vi "datagen 2.vi"() -> ()   [LabVIEW 2020]
uses:
  <vilib>/Graiphic/HAIBAL Deep learning/Source/Layer/Dense/_Controls/dense_param.ctl
  <vilib>/Graiphic/HAIBAL Deep learning/Source/_Controls/activation_enum.ctl
  <vilib>/Graiphic/HAIBAL Deep learning/Source/_Controls/optimizer_param.ctl
  <vilib>/Graiphic/HAIBAL Deep learning/Source/_Controls/optimizer_enum.ctl
  <vilib>/Graiphic/HAIBAL Deep learning/Source/Init/_Controls/Init_Enum.ctl
  <vilib>/Graiphic/HAIBAL Deep learning/Source/Model/Controls/frw_training_mode.ctl
  <vilib>/Graiphic/HAIBAL Deep learning/Source/Layer/Input/_Methods/add_to_graph.vi
  <vilib>/Graiphic/HAIBAL Deep learning/Source/Layer/Dense/_Methods/add_to_graph.vi
  <vilib>/Graiphic/HAIBAL Deep learning/Source/Model/_Methods/summary.vi
  <vilib>/Graiphic/HAIBAL Deep learning/Source/Model/_Methods/mono_input_2d.vi
  <vilib>/Graiphic/HAIBAL Deep learning/Source/Model/_Methods/mono_y_true_2d.vi
  <vilib>/Graiphic/HAIBAL Deep learning/Source/Model/_Methods/backward.vi
  <vilib>/Graiphic/HAIBAL Deep learning/Source/Model/_Methods/get_2d_output_frw.vi
  <vilib>/Graiphic/HAIBAL Deep learning/Source/Layer/Dense/Dense.lvclass
  <vilib>/Graiphic/HAIBAL Deep learning/Source/Model/Model.lvclass
  <vilib>/Graiphic/HAIBAL Deep learning/Source/Layer/Input/Input.lvclass
panel:
  out "Waveform Chart":sgl(graph)
  out "Epoch":i32
  out "Display":cluster{"X":dbl, "Y_True":dbl, "Y_Pred":dbl}[](graph)
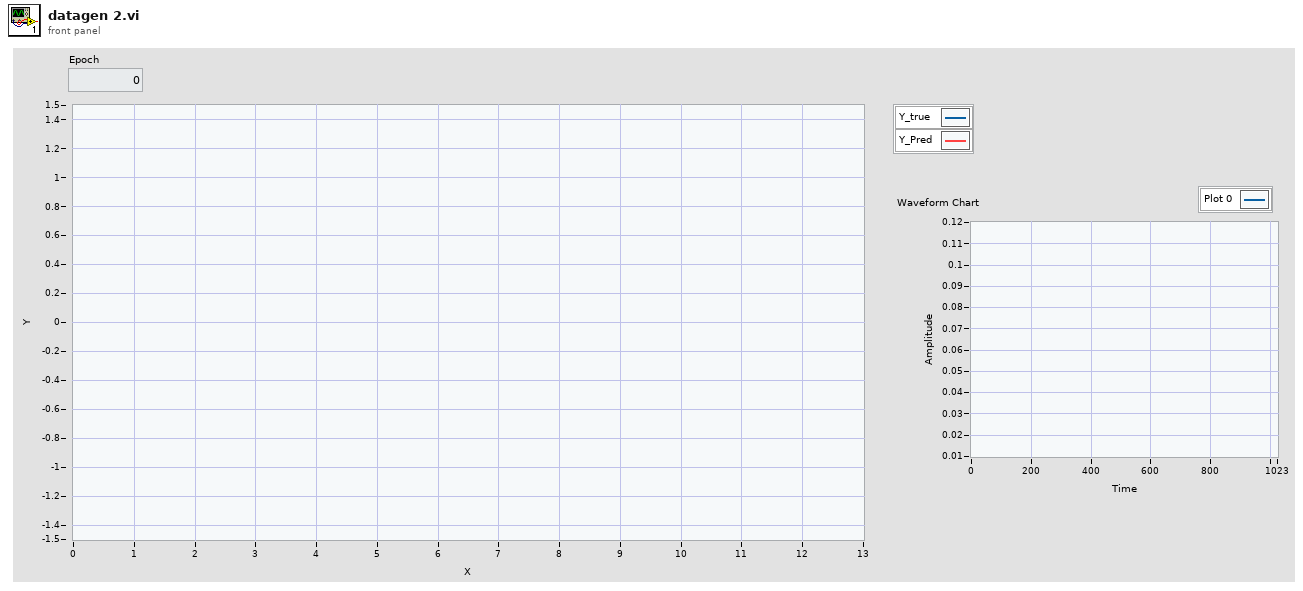
[diagram p1: front panel]
types:
  T1 = typedef "Dense.lvclass/dense_param.ctl" = cluster{"units":i32, "activation":T2, "use_bias?":bool, "optimizer":T3, "weight_initializer":T5, "bias_initializer":T5, "training?":bool, "store?":bool, "update?":bool, "lda_coeff":dbl}
  T2 = typedef "activation_enum.ctl" = enum16{"elu", "exponential", "gelu", "hard_sigmoid", "leaky_relu", "linear", "relu", "selu", "sigmoid", "softmax", "softplus", "softsign", "swish", "tanh", "thresholdedrelu"}
  T3 = typedef "optimizer_param.ctl" = cluster{"algorithm":T4, "learning_rate":sgl, "beta_1":sgl, "beta_2":sgl}
  T4 = typedef "optimizer_enum.ctl" = enum16{"adadelta", "adagrad", "adam", "adamax", "inertia", "nadam", "nesterov", "rmsprop", "sgd"}
  T5 = typedef "Init_Enum.ctl" = enum16{"Constant", "GlorotNormal", "GlorotUniform", "HeNormal", "HeUniform", "Identity", "LeCunNormal", "LeCunUniform", "Ones", "Orthogonal", "RandomNormal", "RandomUniform", "TruncatedNormal", "VarianceScaling", "Zeros"}
  T6 = typedef "frw_training_mode.ctl" = enum16{"Nothing", "Training", "Predict"}
  T7 = typedef "loss_data_cluster.ctl" = cluster{"loss":sgl, "loss_derivate":T8[]}
  T8 = typedef "backward_output_cluster.ctl" = cluster{"name":string, "index":i32, "dimension":T9, "shape":i32[], "data":variant}
  T9 = typedef "loss_der_dimension_enum.ctl" = enum16{"2D Loss Derivate", "3D Loss Derivate", "4D Loss Derivate", "5D Loss Derivate", "6D Loss Derivate"}
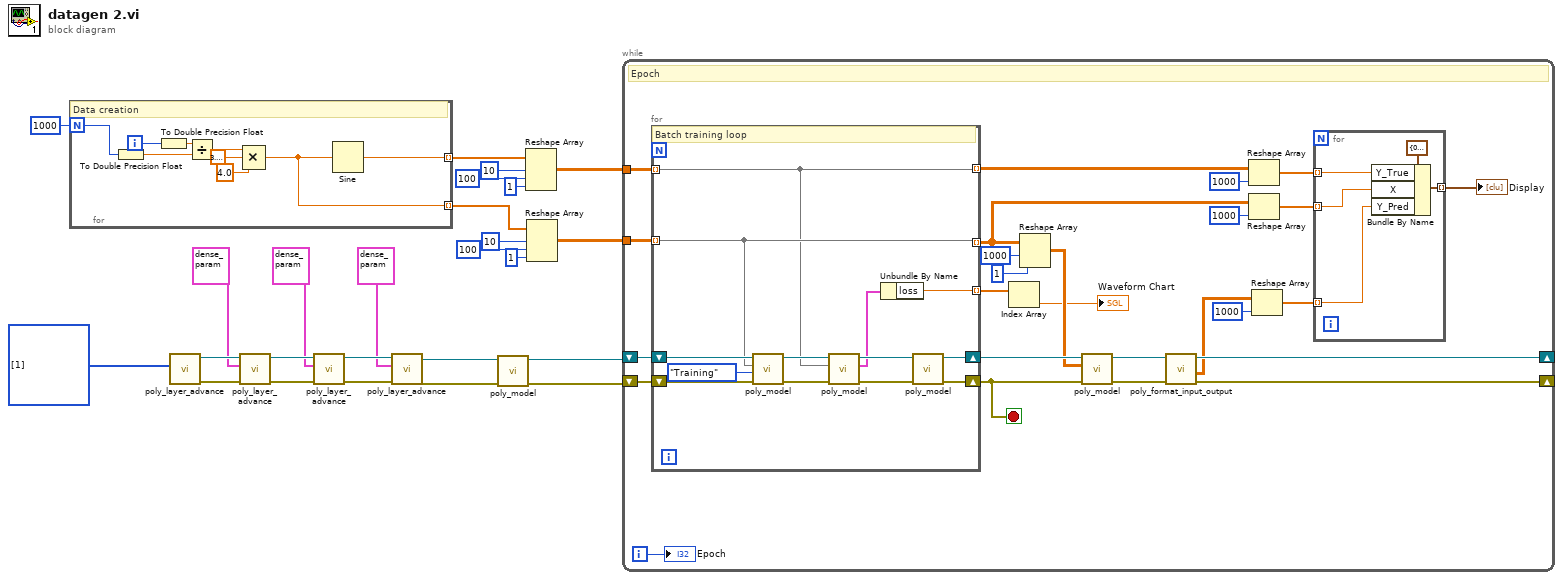
[diagram p0: block diagram]
diagram:
  n1 = for {
    N: 1000 -> [w33]
    tunnel: [w27] -> w14 mode=indexing
    tunnel: [w26] -> w7 mode=indexing
    i -> [w34]
    # "Data creation"
    n2 = To Double Precision Float(number=w33) -> (double precision float=w32:dbl)
    n3 = To Double Precision Float(number=w34) -> (double precision float=w31:dbl)
    n4 = Divide(x=w31, y=w32) -> (x/y=w30:dbl)
    n5 = Compound Arithmetic op=MULTIPLY(w30, 3.141592653589793, 4.0 ("value")) -> (w26:dbl)
    n6 = Sine(x=w26) -> (sin(x)=w27:dbl)
  }
  n7 = call-poly <vilib>:"poly_layer_advance.vi"("input_shape"=i32[] [1]) -> ("error out"=w19:errorcluster, "Graph out"=w20:refnum<class "Model.lvclass">)  [unwired: 9 in]
  n8 = call-poly <vilib>:"poly_layer_advance.vi"("error in"=w19, "parameters"=T1 {"units"=150, "activation"=enum."swish", "use_bias?"=TRUE, "optimizer"={"algorithm"=enum."adam", "learning_rate"=0.001, "beta_1"=0.9, "beta_2"=0.999}, "weight_initializer"=enum."GlorotUniform", "bias_initializer"=enum."Zeros", "training?"=TRUE, "store?"=FALSE, "update?"=TRUE, "lda_coeff"=1.0}, "Graph in"=w20) -> ("error out"=w23:errorcluster, "Graph out"=w24:refnum<class "Model.lvclass">)  [unwired: 7 in]
  n9 = call-poly <vilib>:"poly_layer_advance.vi"("error in"=w23, "parameters"=T1 {"units"=50, "activation"=enum."relu", "use_bias?"=TRUE, "optimizer"={"algorithm"=enum."adam", "learning_rate"=0.001, "beta_1"=0.9, "beta_2"=0.999}, "weight_initializer"=enum."GlorotUniform", "bias_initializer"=enum."Zeros", "training?"=TRUE, "store?"=FALSE, "update?"=TRUE, "lda_coeff"=1.0}, "Graph in"=w24) -> ("error out"=w21:errorcluster, "Graph out"=w22:refnum<class "Model.lvclass">)  [unwired: 7 in]
  n10 = call-poly <vilib>:"poly_layer_advance.vi"("error in"=w21, "parameters"=T1 {"units"=1, "activation"=enum."linear", "use_bias?"=TRUE, "optimizer"={"algorithm"=enum."adam", "learning_rate"=0.001, "beta_1"=0.9, "beta_2"=0.999}, "weight_initializer"=enum."GlorotUniform", "bias_initializer"=enum."Zeros", "training?"=TRUE, "store?"=FALSE, "update?"=TRUE, "lda_coeff"=1.0}, "Graph in"=w22) -> ("error out"=w3:errorcluster, "Graph out"=w4:refnum<class "Model.lvclass">)  [unwired: 7 in]
  n11 = call-poly <vilib>:"poly_model.vi"("error in (no error)"=w3, "Model in"=w4) -> ("error out"=w1:errorcluster, "Model out"=w2:refnum<class "Model.lvclass">)  [unwired: 7 in, 1 out]
  n12 = Reshape Array(w14, 10 ("dimension size"), 100 ("dimension size"), 1 ("dimension size")) -> (w5:dbl[][][])
  n13 = Reshape Array(w7, 10 ("dimension size"), 100 ("dimension size"), 1 ("dimension size")) -> (w6:dbl[][][])
  n14 = while {
    tunnel: w6 -> [w58]
    tunnel: w5 -> [w59]
    shift-right: [w48] -> _
    shift-left: w2 -> [w57]
    shift-right: [w47] -> _
    shift-left: w1 -> [w56]
    i -> [w60]
    stop <- w55 stop-if-true
    # "Epoch"
    n15 = for {
      tunnel: w59 -> [w63] mode=indexing
      tunnel: w58 -> [w64] mode=indexing
      shift-right: [w66] -> w54
      shift-left: w57 -> [w73]
      shift-right: [w65] -> w55
      shift-left: w56 -> [w72]
      tunnel: [w64] -> w43 mode=indexing
      tunnel: [w63] -> w45 mode=indexing
      tunnel: [w61] -> w36 mode=indexing
      # "Batch training loop"
      n16 = call-poly <vilib>:"poly_model.vi"("error in"=w72, "train_mode"=frw_training_mode."Training", "data in"=w64, "Model in"=w73) -> ("error out"=w69:errorcluster, "Model out"=w70:refnum<class "Model.lvclass">)  [unwired: 4 in, 2 out]
      n17 = call-poly <vilib>:"poly_model.vi"("error in"=w69, "y_true_data"=w63, "Model in"=w70) -> ("error out"=w67:errorcluster, "loss_data"=w62:T7, "Model out"=w68:refnum<class "Model.lvclass">)  [unwired: 5 in, 1 out]
      n18 = Unbundle By Name(w62) -> ("loss"=w61:sgl)
      n19 = call-poly <vilib>:"poly_model.vi"("error in"=w67, "Model in"=w68) -> ("error out"=w65:errorcluster, "Model out"=w66:refnum<class "Model.lvclass">)  [unwired: 6 in, 2 out]
    }
    n20 = Index Array(array=w36) -> (element=→"Waveform Chart":sgl)  [unwired: 1 in]
    n21 = Reshape Array(w43, 1000 ("dimension size"), 1 ("dimension size")) -> (w51:dbl[][])
    n22 = call-poly <vilib>:"poly_model.vi"("error in"=w55, "data in"=w51, "Model in"=w54) -> ("error out"=w49:errorcluster, "Model out"=w50:refnum<class "Model.lvclass">)  [unwired: 5 in, 2 out]
    n23 = call-poly <vilib>:"poly_format_input_output.vi"("error in"=w49, "Model in"=w50) -> ("error out"=w47:errorcluster, "output_2d"=w41:sgl[][], "Model out"=w48:refnum<class "Model.lvclass">)  [unwired: 6 in, 1 out]
    n24 = Reshape Array(w45, 1000 ("dimension size")) -> (w38:dbl[])
    n25 = Reshape Array(w43, 1000 ("dimension size")) -> (w39:dbl[])
    n26 = Reshape Array(w41, 1000 ("dimension size")) -> (w40:sgl[])
    n27 = for {
      tunnel: w40 -> [w75] mode=indexing
      tunnel: w39 -> [w76] mode=indexing
      tunnel: w38 -> [w77] mode=indexing
      tunnel: [w74] -> w37 mode=indexing
      n28 = Bundle By Name(cluster=cluster{"X":dbl, "Y_True":dbl, "Y_Pred":dbl} {"X"=0.0, "Y_True"=0.0, "Y_Pred"=0.0}, "Y_True"=w77, "X"=w76, "Y_Pred"=w75) -> (w74:cluster{"X":dbl, "Y_True":dbl, "Y_Pred":dbl})
    }
    "Display" <- w37
    "Epoch" <- w60
  }
